vi "Write Observer Refs.vi"(8 "error in (no error)":errorcluster, 10 "Observer Refs":refnum<queue>[](array[refnum]), 11 "Data Subject in":refnum<class "Data Subject.lvclass">) -> (0 "error out":errorcluster, 3 "Data Subject out":refnum<class "Data Subject.lvclass">)   [LabVIEW 2018, in "Data Subject.lvclass"]
uses:
  Data Subject.lvclass
  Data/Data.lvclass
  Data Subject.lvclass/Data Subject.ctl
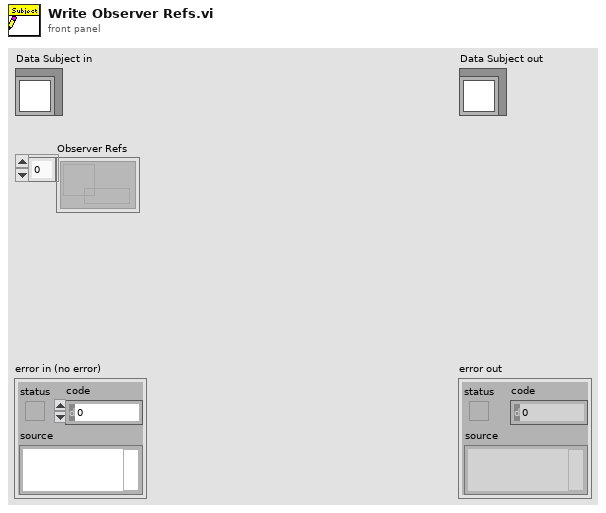
[diagram p1: front panel]
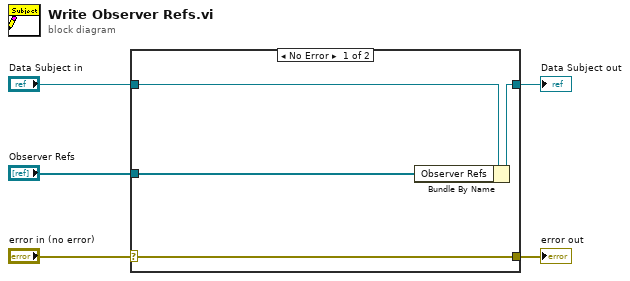
[diagram p0: block diagram]
diagram:
  n1 = case shown="No Error" "error in (no error)" {
    selector: "error in (no error)" -> [w9 w10]
    tunnel: [w9 w10] -> w4
    tunnel: [w7 w11] -> w2
    tunnel: "Data Subject in" -> [w8 w11]
    tunnel: "Observer Refs" -> [w6 _]
    frame No Error {
      n2 = Bundle By Name(cluster=w8, "Observer Refs"=w6) -> (w7:refnum<class "Data Subject.lvclass">)
    }
    frame Error {
    }
  }
  "error out" <- w4
  "Data Subject out" <- w2
